vi "FuturePose.vi"(10 "IA State Input":T1) -> (2 "output cluster":T1={"our_robots"=[], "enemy_robots"=[], "balls"=[], "geometry"={"field_length"=0, "field_width"=0, "goal_width"=0, "goal_depth"=0, "center_circle_radius"=0, "defense_width"=0, "defense_depth"=0, "free_kick_from_defense_dist"=0, "penalty_spot_from_field_line_dist"=0, "penalty_line_from_spot_dist"=0, "half_moon_depth"=0, "half_moon_width"=0}, "IA Judge"={"stage"="", "command"="", "our_goalie_id"=0.0, "enemy_goalie_id"=0.0, "command enum"=enum."Halt", "Time"=enum."Azul"}, "Received Timestamp"=timestamp(0 s since 1904-01-01), "Events"={"Touch"=FALSE, "id touch"=0.0, "Ball out of \nVision"=FALSE, "Ball inside \nGoalie area"=FALSE, "Robot not responding"=FALSE, "Robots responding status"=[1.0, 1.0, 1.0, 1.0, 1.0, 1.0], "Enemy Ball \nPossession"=FALSE, "Id ini Possession"=0.0, "Ball Possesion"=FALSE, "Id Possesion"=0.0, "Ball at\nour goal side"=FALSE, "Ball at\ntouchline"=FALSE, "Ball at\nenemy goal side"=FALSE}})   [LabVIEW 2017]
uses:
  Core/AI Input.ctl
  Core/AI Robot.ctl
  Intel/Functions Enum.ctl
  Intel/AttackerStates.ctl
  Path Planning/RRT/PathDests.ctl
  Path Planning/RRT/PathDest.ctl
  Core/AI Ball.ctl
  Core/Field Size.ctl
  Core/AI Judge.ctl
  Intel/Command Enum.ctl
  Events/Events.ctl
  PreviousState.vi
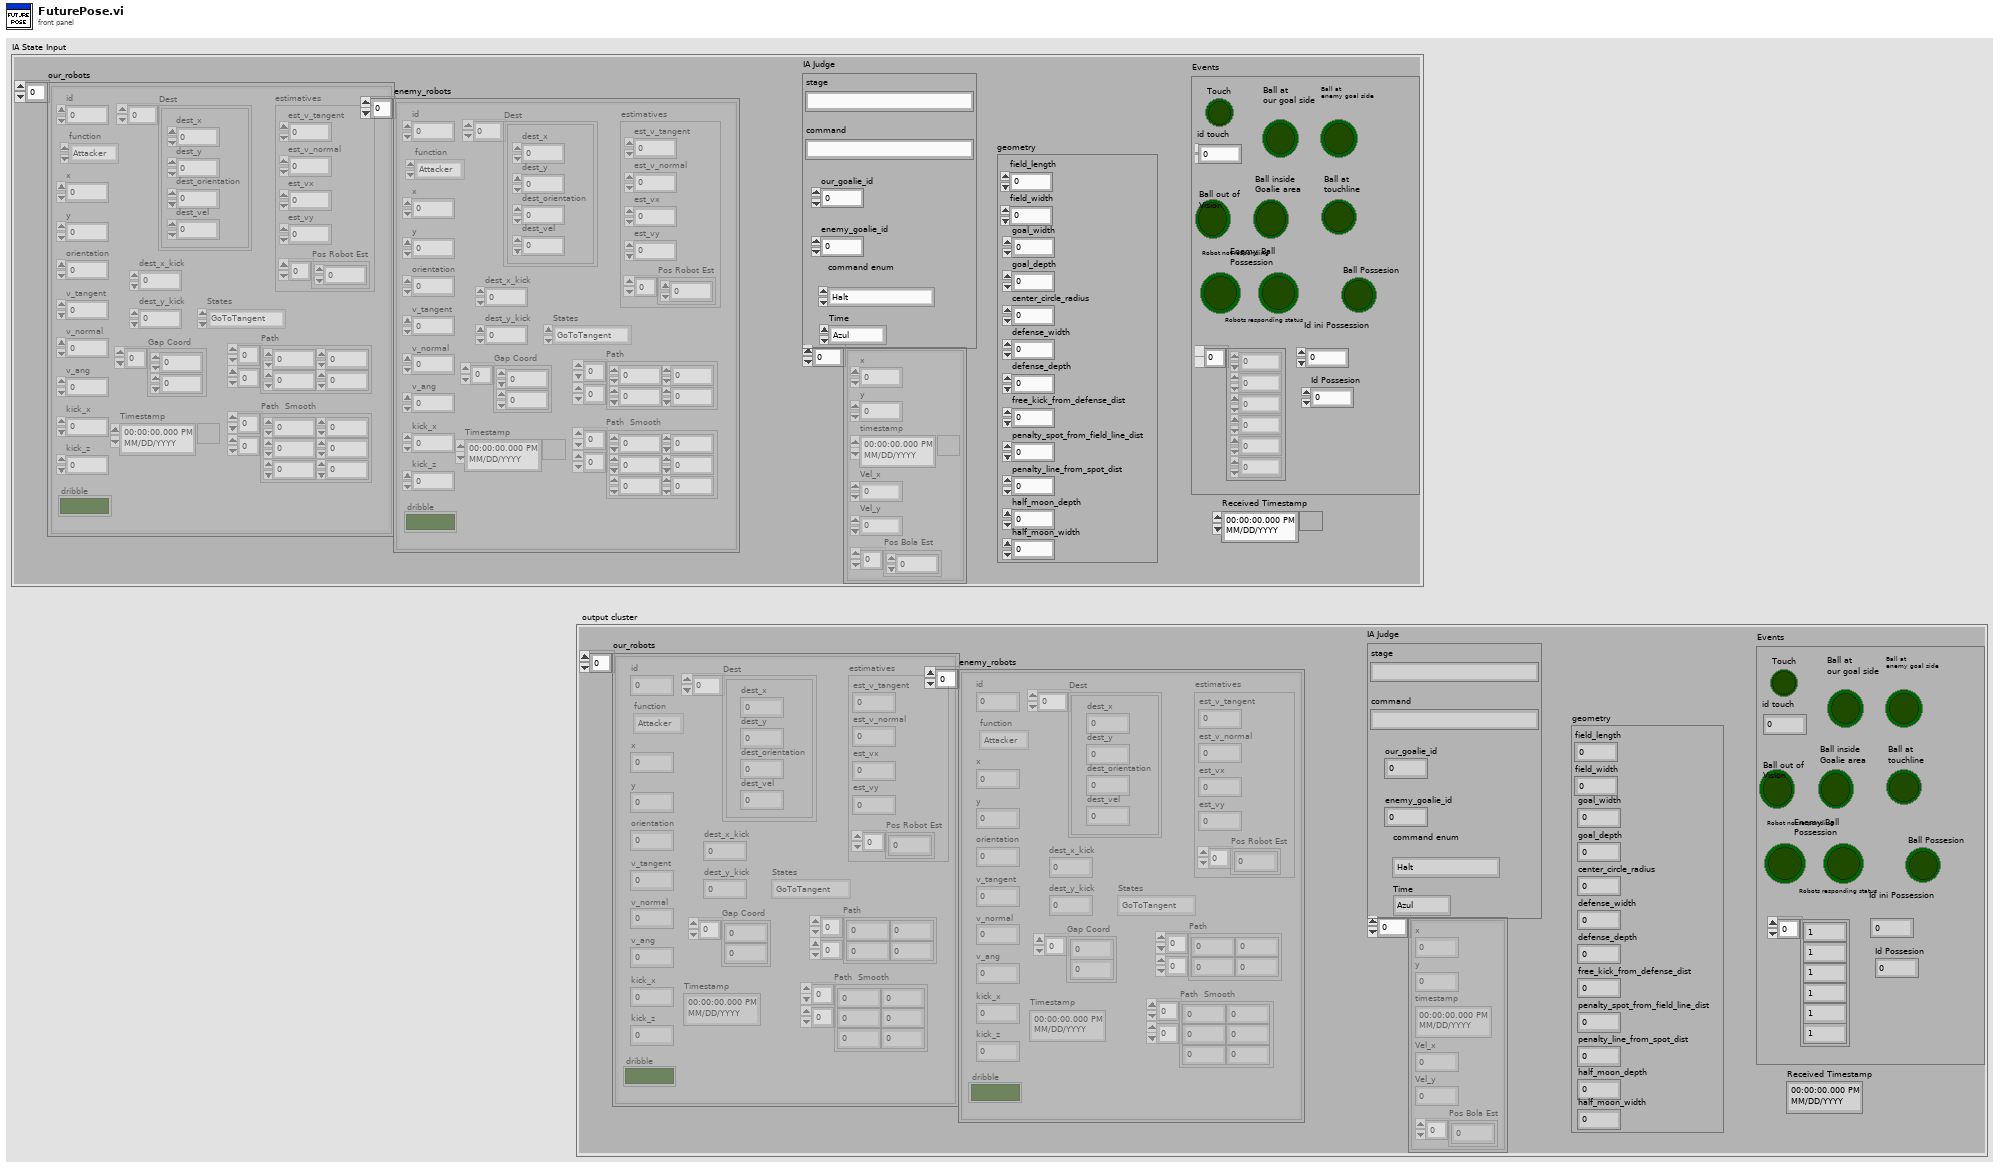
[diagram p1: front panel]
types:
  T1 = typedef "AI Input.ctl" = cluster{"our_robots":T2[], "enemy_robots":T2[], "balls":T7[], "geometry":T8, "IA Judge":T9, "Received Timestamp":timestamp, "Events":T11}
  T2 = typedef "AI Robot.ctl" = cluster{"id":u32, "function":T3, "x":dbl, "y":dbl, "orientation":dbl, "v_tangent":dbl, "v_normal":dbl, "v_ang":dbl, "kick_x":dbl, "kick_z":dbl, "dribble":bool, "Timestamp":timestamp, "estimatives":cluster{"est_v_tangent":dbl, "est_v_normal":dbl, "est_vx":dbl, "est_vy":dbl, "Pos Robot Est":dbl[]}, "dest_x_kick":dbl, "dest_y_kick":dbl, "Gap Coord":dbl[], "States":T4, "Path ":dbl[][], "Path  Smooth":dbl[][], "Dest":T5}
  T3 = typedef "Functions Enum.ctl" = enum16{"Attacker", "Goalie", "Defender", "Striker", "Goto 0", "Dummy", "Kicker", "ZigZag"}
  T4 = typedef "AttackerStates.ctl" = enum16{"Pass", "GoToTangent", "BallGetting", "GoToKick", "Rotate anti-clockwise", "Rotate Clockwise", ""}
  T5 = typedef "PathDests.ctl" = T6[]
  T6 = typedef "PathDest.ctl" = cluster{"dest_x":dbl, "dest_y":dbl, "dest_orientation":dbl, "dest_vel":dbl}
  T7 = typedef "AI Ball.ctl" = cluster{"x":dbl, "y":dbl, "timestamp":timestamp, "Vel_x":dbl, "Vel_y":dbl, "Pos Bola Est":dbl[]}
  T8 = typedef "Field Size.ctl" = cluster{"field_length":u32, "field_width":u32, "goal_width":u32, "goal_depth":u32, "center_circle_radius":u32, "defense_width":u32, "defense_depth":u32, "free_kick_from_defense_dist":u32, "penalty_spot_from_field_line_dist":u32, "penalty_line_from_spot_dist":u32, "half_moon_depth":u32, "half_moon_width":u32}
  T9 = typedef "AI Judge.ctl" = cluster{"stage":string, "command":string, "our_goalie_id":dbl, "enemy_goalie_id":dbl, "command enum":T10, "Time":enum16{"Azul", "Amarelo"}}
  T10 = typedef "Command Enum.ctl" = enum16{"Halt", "Stop", "Force Start", "PKA Normal Start", "Prepare Kickoff Ally", "PKE Normal Start", "Prepare Kickoff Enemy", "Prepare Penalty Ally", "PPA Normal Start", "Prepare Penalty Enemy", "PPE Normal Start", "Direct Free Enemy", "Direct Free Ally", "Indirect Free Enemy", "Indirect Free Ally", "Timeout Enemy", "Timeout Ally", "Goal Enemy", "Goal Ally", "Ball Placement Enemy", "Ball Placement Ally", "Normal Half Time", "Extra Time Break", "Extra Half Time", "None", "Post Game"}
  T11 = typedef "Events.ctl" = cluster{"Touch":bool, "id touch":dbl, "Ball out of \nVision":bool, "Ball inside \nGoalie area":bool, "Robot not responding":bool, "Robots responding status":dbl[], "Enemy Ball \nPossession":bool, "Id ini Possession":dbl, "Ball Possesion":bool, "Id Possesion":dbl, "Ball at\nour goal side":bool, "Ball at\ntouchline":bool, "Ball at\nenemy goal side":bool}
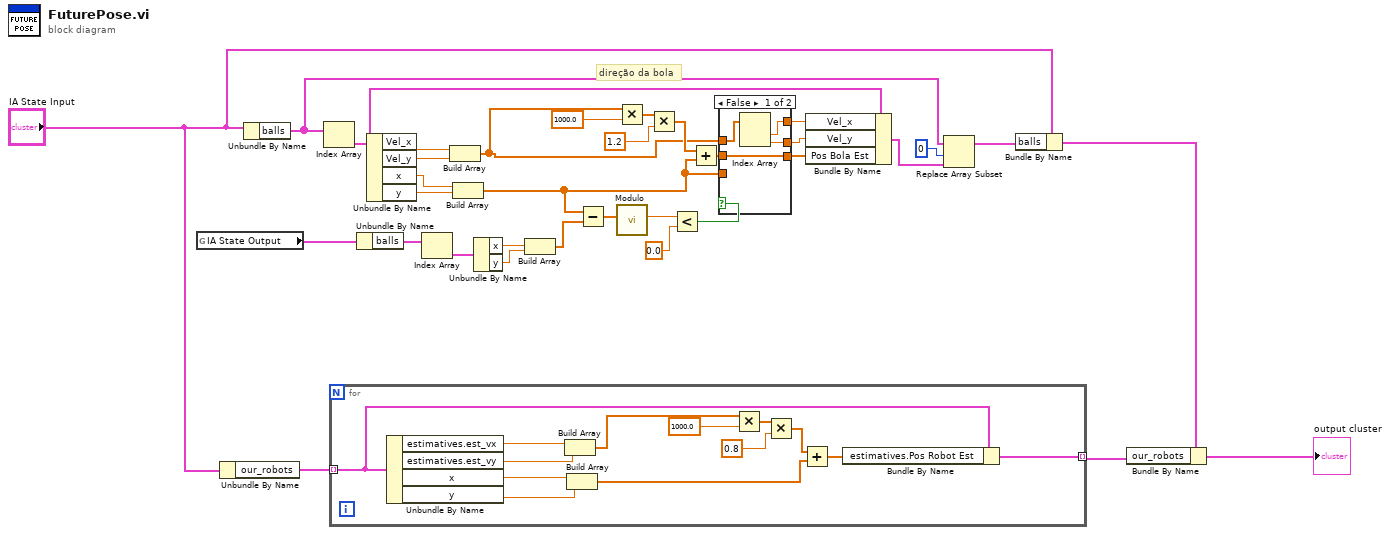
[diagram p0: block diagram]
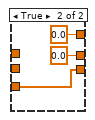
[diagram p2: hidden frame]
diagram:
  # "direção da bola"
  n1 = global read "PreviousState.vi" "IA State Output"() -> (w16:T1)
  n2 = Unbundle By Name("IA State Input") -> ("our_robots"=w20:T2[])
  n3 = Unbundle By Name("IA State Input") -> ("balls"=w30:T7[])
  n4 = Index Array(array=w30) -> (element=w32:T7)  [unwired: 1 in]
  n5 = for {
    tunnel: w20 -> [w37] mode=indexing
    tunnel: [w35] -> w17 mode=indexing
    n6 = Unbundle By Name(w37) -> ("estimatives.est_vx"=w41:dbl, "estimatives.est_vy"=w40:dbl, "x"=w39:dbl, "y"=w38:dbl)
    n7 = Build Array(w41, w40) -> (w43:dbl[])
    n8 = Build Array(w39, w38) -> (w42:dbl[])
    n9 = Multiply(x=w43, y=1000.0) -> (x*y=w45:dbl[])
    n10 = Multiply(x=w45, y=0.8) -> (x*y=w46:dbl[])
    n11 = Add(x=w46, y=w42) -> (x+y=w36:dbl[])
    n12 = Bundle By Name(cluster=w37, "estimatives.Pos Robot Est"=w36) -> (w35:T2)
  }
  n13 = Unbundle By Name(w16) -> ("balls"=w15:T7[])
  n14 = Unbundle By Name(w32) -> ("Vel_x"=w34:dbl, "Vel_y"=w33:dbl, "x"=w27:dbl, "y"=w26:dbl)
  n15 = Index Array(array=w15) -> (element=w14:T7)  [unwired: 1 in]
  n16 = Build Array(w34, w33) -> (w3:dbl[])
  n17 = Build Array(w27, w26) -> (w4:dbl[])
  n18 = Unbundle By Name(w14) -> ("x"=w11:dbl, "y"=w10:dbl)
  n19 = Build Array(w11, w10) -> (w9:dbl[])
  n20 = Subtract(x=w4, y=w9) -> (x-y=w8:dbl[])
  n21 = Multiply(x=w3, y=1000.0) -> (x*y=w24:dbl[])
  n22 = call "Modulo.vi"("2D vector"=w8) -> ("Modulo"=w7:dbl)  [unwired: 10 in]
  n23 = Multiply(x=w24, y=1.2) -> (x*y=w23:dbl[])
  n24 = Less?(x=w7, y=0.0) -> (x < y?=w5:bool)
  n25 = Add(x=w23, y=w4) -> (x+y=w13:dbl[])
  n26 = case shown="False" w5 {
    tunnel: [w51 w54] -> w12
    tunnel: w13 -> [w51 _]
    tunnel: w4 -> [_ w54]
    tunnel: w3 -> [w50 _]
    tunnel: [w49 0.0 ("Vel_y")] -> w2
    tunnel: [w48 0.0 ("Vel_y")] -> w1
    frame False {
      n27 = Index Array(array=w50) -> (element #1=w49:dbl, element #2=w48:dbl)  [unwired: 2 in]
    }
    frame True {
    }
  }
  n28 = Bundle By Name(cluster=w32, "Vel_x"=w2, "Vel_y"=w1, "Pos Bola Est"=w12) -> (w29:T7)
  n29 = Replace Array Subset(array=w30, new element=w29, index=0) -> (w31:T7[])
  n30 = Bundle By Name(cluster="IA State Input", "balls"=w31) -> (w19:T1)
  n31 = Bundle By Name(cluster=w19, "our_robots"=w17) -> (→"output cluster":T1)
